vi "NicmosWriteMaskBanks.vi"(3 "refnum in":T1, 9 "error in (no error)":errorcluster) -> (0 "refnum out":T1, 6 "error out":errorcluster)   [LabVIEW 2009]
uses:
  <vilib>/Utility/config.llb/Config Data RefNum.ctl
  <vilib>/Utility/config.llb/NI_LVConfig.lvlib
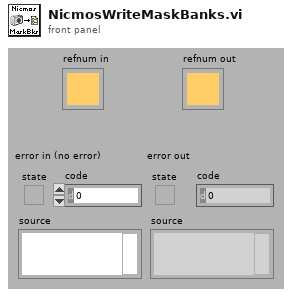
[diagram p1: front panel]
types:
  T1 = typedef "NI_LVConfig.lvlib/Config Data RefNum.ctl" = refnum<k1>
  T2 = typedef "NICMOS.MASKBANKS.ctl" = cluster{"MaskList":cluster{"X":i32, "Y":i32, "NX":i32, "NY":i32}[], "Reform X":i32, "Reform Y":i32}[]
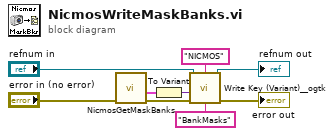
[diagram p0: block diagram]
diagram:
  n1 = call "NicmosGetMaskBanks.vi"("error in (no error)"="error in (no error)") -> ("READOUT out"=w1:T2, "error out"=w2:errorcluster)  [unwired: 7 in]
  n2 = To Variant(anything=w1) -> (Variant=w9:variant)
  n3 = call <userlib>:"Write Key (Variant)__ogtk.vi"("section"="NICMOS", "error in (no error)"=w2, "key-value"=w9, "key (optional)"="BankMasks", "refnum"="refnum in") -> ("error out"=→"error out":errorcluster, "refnum out"=→"refnum out":T1)  [unwired: 5 in]
